vi "Polynomial Remove Trailing Zeros.vi"(10 "Coefficients":dbl[](array[numeric])) -> (2 "Used Coefficients":dbl[](array[numeric]))   [LabVIEW 2020, in "VolatusData.lvlib" / "Scaling.lvclass"]
uses:
  Scaling.lvclass
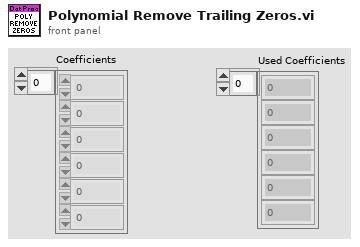
[diagram p1: front panel]
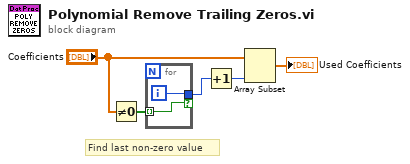
[diagram p0: block diagram]
diagram:
  # "Find last non-zero value"
  n1 = Not Equal To 0?(x="Coefficients") -> (x != 0?=w5:bool[])
  n2 = for {
    tunnel: w5 -> [w6] mode=indexing
    tunnel: [w7] -> w3 if=w6
    i -> [w7]
  }
  n3 = Increment(x=w3) -> (x+1=w2:i32)
  n4 = Array Subset(array="Coefficients", length=w2) -> (→"Used Coefficients":dbl[])  [unwired: 1 in]
